vi "ConfigureHighRateVibrationAnalysis.vi"(8 "error in (no error)":errorcluster) -> (0 "error out":errorcluster, 2 "register trends":T1[](array[typedef]), 3 "analysis config":T3, 5 "valid config":bool)   [LabVIEW 2017, in "CmsAnalysisHighRate.lvlib"]
uses:
  <vilib>/addons/InsightCM/Devices/Shared/Cms/CmsAnalysisHighRate/CmsAnalysisHighRate.lvlib
  <vilib>/addons/InsightCM/Devices/Shared/Cms/CmsAnalysis/controls/Config.ctl
  <vilib>/addons/InsightCM/Devices/Shared/Cms/CmsAnalysis/controls/Group.ctl
  <vilib>/addons/InsightCM/Utilities/Analysis/Shared/controls/Channel.ctl
  <vilib>/addons/InsightCM/Utilities/Analysis/Shared/controls/SpeedType.ctl
  <vilib>/addons/InsightCM/Utilities/Analysis/Shared/controls/Feature.ctl
  <vilib>/addons/InsightCM/Utilities/Analysis/Shared/controls/AmplitudeScale.ctl
  <vilib>/addons/InsightCM/Devices/Shared/Common/DataEventCreator/controls/RegisterTrendPoints.ctl
  <vilib>/addons/InsightCM/Devices/Shared/Common/DataEventCreator/controls/Registry_Trend.ctl
  <vilib>/addons/InsightCM/Utilities/Analysis/Shared/AnalysisHelper.lvlib
  <vilib>/addons/InsightCM/Utilities/GlobalConfiguration/GlobalConfiguration.lvlib
  <vilib>/addons/InsightCM/Utilities/DeviceModelHelpers/DeviceModelHelpers.lvlib
  <vilib>/addons/InsightCM/Devices/Shared/Cms/CmsAnalysis/CmsAnalysis.lvlib
  <vilib>/addons/InsightCM/Utilities/PropertyHelpers/PropertyHelpers.lvlib
  <vilib>/addons/InsightCM/Devices/Shared/Cms/CmsVirtualChannel/CmsVirtualChannel.lvlib
  <vilib>/addons/InsightCM/Devices/Shared/Common/DataEventCreator/DataEventCreator.lvlib
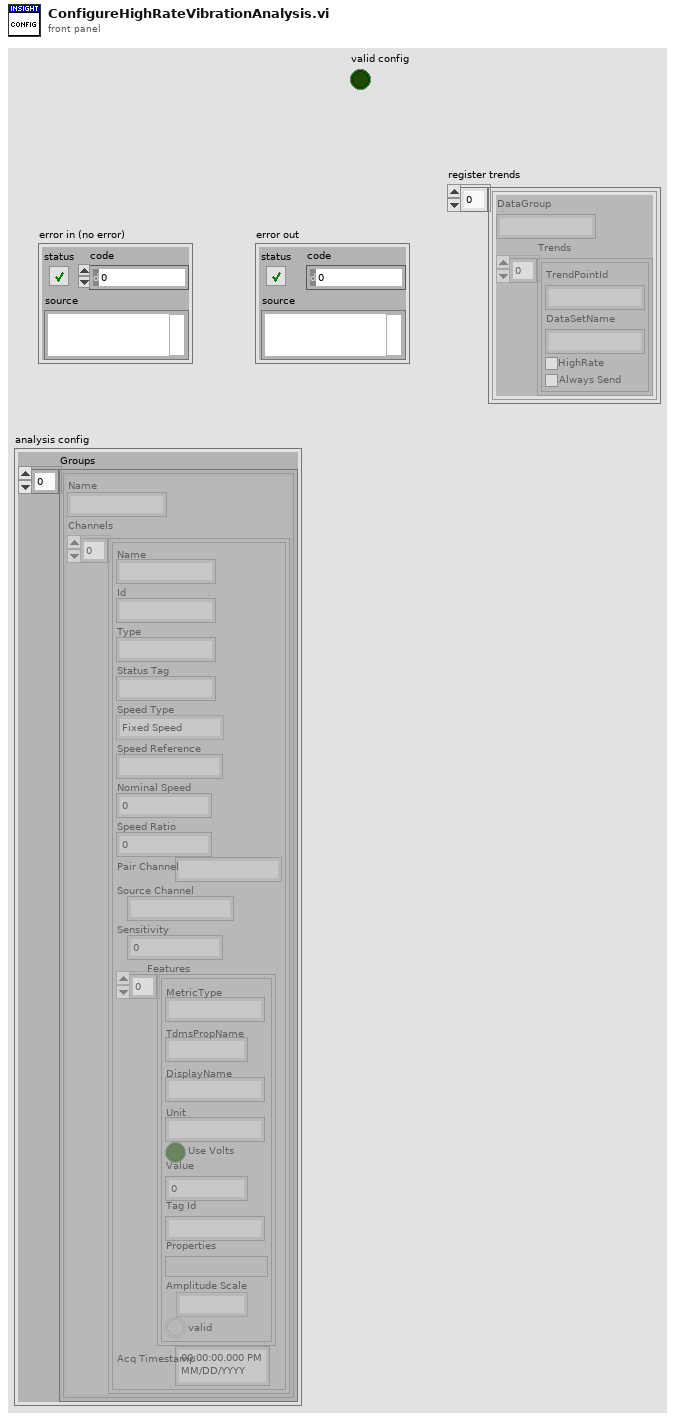
[diagram p1: front panel]
types:
  T1 = typedef "DataEventCreator.lvlib/RegisterTrendPoints.ctl" = cluster{"DataGroup":string, "Trends":T2[]}
  T2 = typedef "DataEventCreator.lvlib/Registry_Trend.ctl" = cluster{"TrendPointId":string, "DataSetName":string, "HighRate":bool, "Always Send":bool}
  T3 = typedef "CmsAnalysis.lvlib/Config.ctl" = cluster{"Groups":T4[]}
  T4 = typedef "CmsAnalysis.lvlib/Group.ctl" = cluster{"Name":string, "Channels":T5[]}
  T5 = typedef "AnalysisHelper.lvlib/Channel.ctl" = cluster{"Name":string, "Id":string, "Type":string, "Status Tag":string, "Speed Type":T6, "Speed Reference":string, "Nominal Speed":dbl, "Speed Ratio":dbl, "Pair Channel":string, "Source Channel":string, "Sensitivity":dbl, "Features":T7[], "Acq Timestamp":timestamp}
  T6 = typedef "AnalysisHelper.lvlib/SpeedType.ctl" = enum16{"Fixed Speed", "Tachometer", "From Map"}
  T7 = typedef "AnalysisHelper.lvlib/Feature.ctl" = cluster{"MetricType":string, "TdmsPropName":string, "DisplayName":string, "Unit":string, "Use Volts":bool, "Value":dbl, "Tag Id":string, "Properties":variant, "Amplitude Scale":T8, "valid":bool}
  T8 = typedef "AnalysisHelper.lvlib/AmplitudeScale.ctl" = enum16{"rms", "peak", "pk-pk"}
  T9 = typedef "R2_DeviceModel.ctl" = cluster{"Device":T10, "Channels":T18[], "Tags":T20[]}
  T10 = typedef "R2_Device.ctl" = cluster{"Id":string, "Name":string, "DeviceType":string, "HardwareName":string, "IpAddress":string, "HardwareInfo":T11[], "ApplicationType":string, "ApplicationVersion":string, "EquipmentIds":string[], "ConfigurationVersion":string, "State":T12, "Properties":T11[], "DataGroups":T13[], "BurstModeTrigger":T17}
  T11 = typedef "KeyValuePair.ctl" = cluster{"Key":string, "Value":string}
  T12 = typedef "DeviceState.ctl" = cluster{"Disabled":bool}
  T13 = typedef "R2_DataGroup.ctl" = cluster{"Name":string, "OperatingStates":T14[], "Properties":T11[], "EquipmentIds":string[], "AssetNodeId":string}
  T14 = typedef "OperatingState.ctl" = cluster{"Name":string, "Properties":T11[], "Triggers":T15[]}
  T15 = typedef "Trigger.ctl" = cluster{"Type":string, "Expression":string, "Conditions":T16[]}
  T16 = typedef "Condition.ctl" = cluster{"Source":string, "Type":string, "Operator":string, "CompareTo":string, "DwellSeconds":dbl}
  T17 = typedef "BurstModeTrigger.ctl" = cluster{"Trigger":T15, "SampleRate":string, "AcquisitionLength":string}
  T18 = typedef "R2_Channel.ctl" = cluster{"Id":string, "DeviceId":string, "Name":string, "ChannelType":string, "HardwareKey":string, "HardwareChannel":string, "DataGroup":string, "Keywords":string[], "EquipmentIds":string[], "Properties":T11[], "Metrics":T19[], "AssetNodeId":string, "MeasType":string, "AssetName":string}
  T19 = typedef "Metric.ctl" = cluster{"Id":string, "Name":string, "Unit":string, "Properties":T11[], "MetricDefinitionInstanceId":string}
  T20 = typedef "Tag.ctl" = cluster{"Id":string, "Path":string, "Name":string, "Datatype":string, "Props":T11[], "Keywords":string[]}
  T21 = typedef "SectionKeyValues.ctl" = cluster{"Section":string, "KeyValues":T11[]}
  T22 = typedef "MetricDefinitionInstance.ctl" = cluster{"Id":string, "MetricType":string, "Name":string, "Properties":T11[], "HighRate":bool}
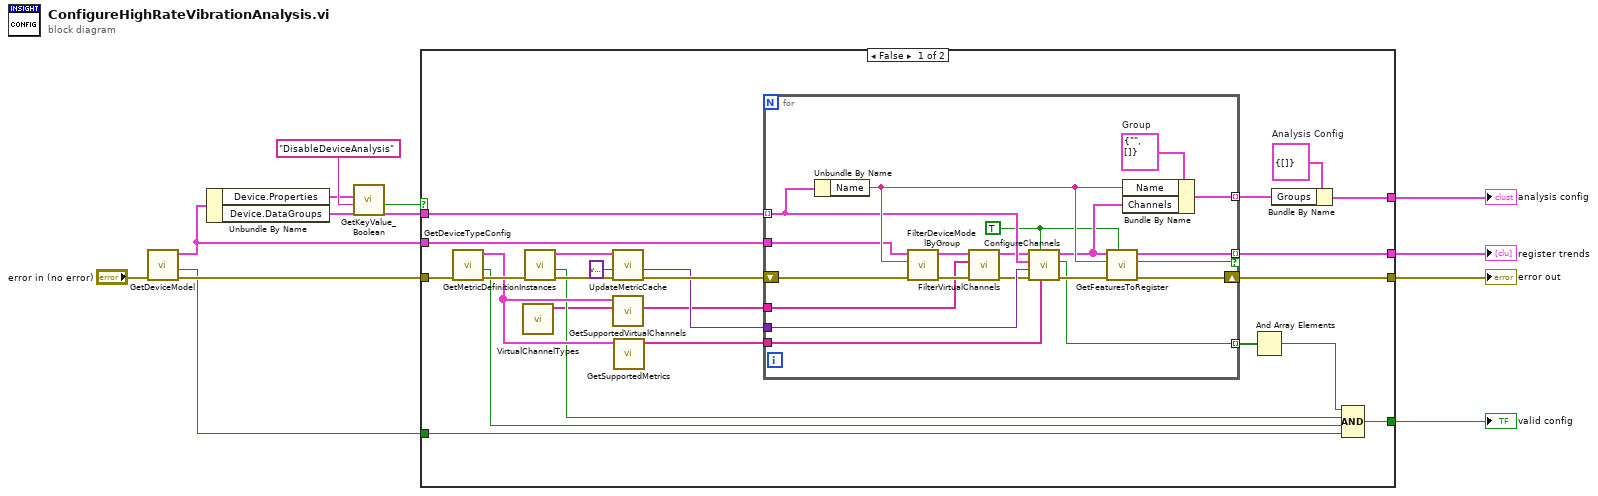
[diagram p0: block diagram]
diagram:
  n1 = call <vilib>:"GetDeviceModel.vi"("error in (no error)"="error in (no error)") -> ("error out"=w7:errorcluster, "found"=w2:bool, "device model"=w6:T9)  [unwired: 8 in]
  n2 = Unbundle By Name(w6) -> ("Device.Properties"=w4:T11[], "Device.DataGroups"=w12:T13[])
  n3 = call <vilib>:"GetKeyValue_Boolean.vi"("key"="DisableDeviceAnalysis", "key value pairs"=w4) -> ("value"=w3:bool)  [unwired: 7 in, 2 out]
  n4 = case shown="False" w3 {
    tunnel: w12 -> [w36 _]
    tunnel: [w35 w58] -> w11
    tunnel: [w34 _] -> w10
    tunnel: [w33 _] -> w9
    tunnel: w7 -> [w32 w58]
    tunnel: w6 -> [w31 _]
    tunnel: w2 -> [w18 w57]
    tunnel: [w14 w57] -> w1
    frame False {
      w25 = T3 {"Groups"=[]}  # Analysis Config
      n5 = call <vilib>:"GetDeviceTypeConfig.vi"("error in (no error)"=w32) -> ("error out"=w23:errorcluster, "found"=w19:bool, "key values"=w22:T21[])  [unwired: 8 in]
      n6 = call <vilib>:"VirtualChannelTypes.vi"() -> ("Array"=w13:string[])  [unwired: 11 in]
      n7 = call <vilib>:"GetMetricDefinitionInstances.vi"("error in (no error)"=w23) -> ("error out"=w30:errorcluster, "found"=w16:bool, "metrics"=w28:T22[])  [unwired: 8 in]
      n8 = call <vilib>:"UpdateMetricCache.vi"("error in (no error)"=w30, "Metrics"=variant, "MetricDefinitionInstances"=w28) -> ("error out"=w29:errorcluster, "Metrics out"=w27:variant)  [unwired: 7 in]
      n9 = call <vilib>:"GetSupportedVirtualChannels.vi"("default virtual channel types"=w13, "key values"=w22) -> ("not supported virtual channels"=w21:string[])  [unwired: 9 in]
      n10 = call <vilib>:"GetSupportedMetrics.vi"("key values"=w22) -> ("supported metrics"=w20:string[])  [unwired: 10 in]
      n11 = for {
        tunnel: w27 -> [w56]
        tunnel: w31 -> [w39]
        shift-right: [w53] -> w35
        shift-left: w29 -> [w54]
        tunnel: [w55] -> w24 mode=indexing
        tunnel: w36 -> [w48] mode=indexing
        tunnel: [w52] -> w34 mode=indexing if=w51
        tunnel: w20 -> [w47]
        tunnel: w21 -> [w40]
        tunnel: [w37] -> w17 mode=indexing
        w38 = TRUE ("high rate")
        w49 = T4 {"Name"="", "Channels"=[]}  # Group
        n12 = Unbundle By Name(w48) -> ("Name"=w50:string)
        n13 = call <vilib>:"FilterDeviceModelByGroup.vi"("error in (no error)"=w54, "group"=w50, "device model"=w39) -> ("error out"=w41:errorcluster, "device model (channels filtered by group)"=w43:T9)  [unwired: 7 in]
        n14 = call <vilib>:"FilterVirtualChannels.vi"("error in (no error)"=w41, "not supported virtual channels"=w40, "device model"=w43) -> ("error out"=w42:errorcluster, "device model (unsupported virtual channels filtered out)"=w44:T9)  [unwired: 7 in]
        n15 = call <vilib>:"ConfigureChannels.vi"("supported metrics"=w47, "high rate"=w38, "error in (no error)"=w42, "metric cache"=w56, "group"=w48, "device"=w44) -> ("error out"=w45:errorcluster, "valid config"=w37:bool, "channels"=w46:T5[])  [unwired: 3 in]
        n16 = call <vilib>:"GetFeaturesToRegister.vi"("high rate"=w38, "error in (no error)"=w45, "group"=w50, "channels"=w46) -> ("error out"=w53:errorcluster, "atleast one"=w51:bool, "register trend"=w52:T1)  [unwired: 5 in]
        n17 = Bundle By Name(cluster=w49, "Name"=w50, "Channels"=w46) -> (w55:T4)
      }
      n18 = And Array Elements(Boolean array=w17) -> (logical AND=w15:bool)
      n19 = Bundle By Name(cluster=w25, "Groups"=w24) -> (w33:T3)
      n20 = Compound Arithmetic op=AND(w15, w16, w19, w18) -> (w14:bool)
    }
    frame True {
    }
  }
  "error out" <- w11
  "analysis config" <- w9
  "register trends" <- w10
  "valid config" <- w1
